vi "Add Member Actual Attendance To Dict.vi"(6 "AttendRecord.lvclass":refnum<class "AttendRecord.lvclass">, 8 "error in (no error)":errorcluster, 9 "Name(\"\")":string, 10 "Department(\"\")":string, 11 "CalAttendance in":refnum<class "CalAttendance.lvclass">) -> (0 "error out":errorcluster, 3 "CalAttendance out":refnum<class "CalAttendance.lvclass">)   [LabVIEW 2015, in "CalAttendance.lvclass"]
uses:
  CalAttendance.lvclass
  Models/Attendance Record/AttendRecord.lvclass
  CalAttendance.lvclass/CalAttendance.ctl
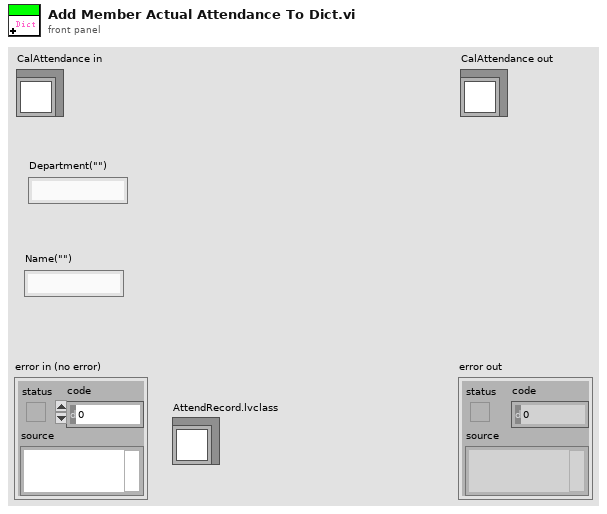
[diagram p1: front panel]
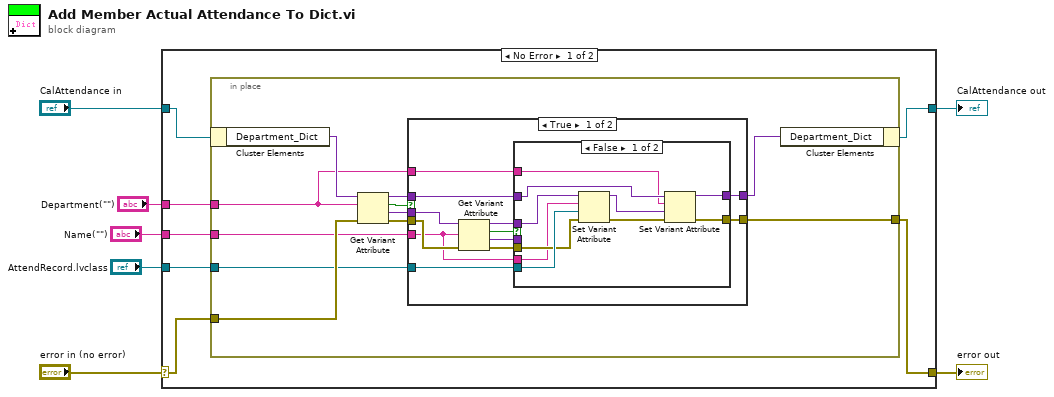
[diagram p0: block diagram]
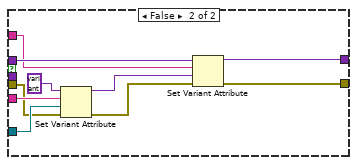
[diagram p3: hidden frame]
diagram:
  n1 = case shown="No Error" "error in (no error)" {
    selector: "error in (no error)" -> [w12 w61]
    tunnel: [w8 w61] -> w6
    tunnel: [w9 w60] -> w4
    tunnel: "CalAttendance in" -> [w14 w60]
    tunnel: "Name(\"\")" -> [w11 _]
    tunnel: "Department(\"\")" -> [w13 _]
    tunnel: "AttendRecord.lvclass" -> [w10 _]
    frame No Error {
      n2 = in-place {
        in-place-border: w13 -> [w17]
        in-place-border: w12 -> [w22]
        in-place-border: w11 -> [w21]
        in-place-border: w10 -> [w20]
        in-place-border: [w15] -> w8
        n3 = in-place-cluster #1(w14) -> ("Department_Dict"=w25:variant)
        n4 = Get Variant Attribute(Variant=w25, name=w17, error in=w22) -> (duplicate Variant=w23:variant, found=w24:bool, value=w19:variant, error out=w18:errorcluster)  [unwired: 1 in]
        n5 = case shown="True" w24 {
          tunnel: w23 -> [w27 w56]
          tunnel: w21 -> [w26 w59]
          tunnel: w20 -> [w29 w58]
          tunnel: w19 -> [w34 _]
          tunnel: w18 -> [w33 w57]
          tunnel: w17 -> [w37 w55]
          tunnel: [w36 w52] -> w15
          tunnel: [w35 w51] -> w16
          frame True {
            n6 = Get Variant Attribute(Variant=w34, name=w26, error in=w33) -> (duplicate Variant=w28:variant, found=w32:bool, value=w31:variant, error out=w30:errorcluster)  [unwired: 1 in]
            n7 = case shown="False" w32 {
              tunnel: w27 -> [w42 w49]
              tunnel: w37 -> [w40 _]
              tunnel: [w44 w48] -> w36
              tunnel: [w38 w49] -> w35
              tunnel: w31 -> [_ _]
              tunnel: w30 -> [w46 w48]
              tunnel: w29 -> [w47 _]
              tunnel: w28 -> [w45 _]
              tunnel: w26 -> [w41 _]
              frame False {
                n8 = Set Variant Attribute(Variant=w45, name=w41, value=w47, error in=w46) -> (Variant out=w39:variant, error out=w43:errorcluster)  [unwired: 1 out]
                n9 = Set Variant Attribute(Variant=w42, name=w40, value=w39, error in=w43) -> (Variant out=w38:variant, error out=w44:errorcluster)  [unwired: 1 out]
              }
              frame True {
              }
            }
          }
          frame False {
            n10 = Set Variant Attribute(Variant=variant ("variant"), name=w59, value=w58, error in=w57) -> (Variant out=w54:variant, error out=w53:errorcluster)  [unwired: 1 out]
            n11 = Set Variant Attribute(Variant=w56, name=w55, value=w54, error in=w53) -> (Variant out=w51:variant, error out=w52:errorcluster)  [unwired: 1 out]
          }
        }
        n12 = in-place-cluster #1("Department_Dict"=w16) -> (w9:refnum<class "CalAttendance.lvclass">)
      }
    }
    frame Error {
    }
  }
  "error out" <- w6
  "CalAttendance out" <- w4
